vi "ROS_Read_Cam.vi"(8 "error in (no error)":errorcluster, 11 "ROS in":T1) -> (0 "error out":errorcluster, 2 "number":u8[](array[numeric]), 3 "Header":T3)   [LabVIEW 2017]
uses:
  <vilib>/Tufts CEEO ROS for LabVIEW Software/ROS/Code/SubVIs/_ROSControl.ctl
  <vilib>/Tufts CEEO ROS for LabVIEW Software/ROS/Code/SubVIs/_ROSDirection.ctl
  <vilib>/Tufts CEEO ROS for LabVIEW Software/ROS/MessageParsing/std_msgs/subs/parse_string_scalar.vi
  <vilib>/Tufts CEEO ROS for LabVIEW Software/ROS/MessageParsing/std_msgs/subs/parse_u8_array.vi
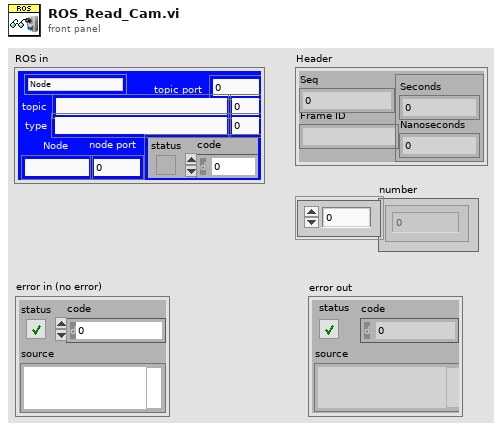
[diagram p1: front panel]
types:
  T1 = typedef "_ROSControl.ctl" = cluster{"topic port":u16, "Node":string, "topic":string, "type":string, "node port":u16, "error ":errorcluster, "Direction":T2, "Update (ms)":u16, "FIFO size":u16}
  T2 = typedef "_ROSDirection.ctl" = enum16{"Node", "Publisher", "Subscriber", "ServiceClient", "ServiceProvider"}
  T3 = cluster{"Seq":u32, "Frame ID":string, "Timestamp":cluster{"Seconds":i32, "Nanoseconds":i32}}
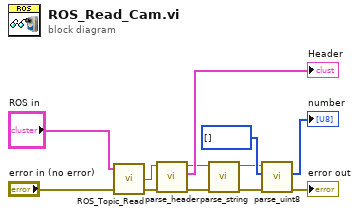
[diagram p0: block diagram]
diagram:
  n1 = call <vilib>:"ROS_Topic_Read.vi"("error in (no error)"="error in (no error)", "ROS in"="ROS in") -> ("error out"=w4:errorcluster, "Reply"=w5:string)  [unwired: 1 in, 1 out]
  n2 = call <vilib>:"parse_header.vi"("error in"=w4, "msg in"=w5) -> ("error out"=w3:errorcluster, "Header"=→"Header":T3, "msg out"=w6:string)  [unwired: 3 in]
  n3 = call-poly <vilib>:"parse_string.vi"("error in"=w3, "msg in"=w6) -> ("error out"=w2:errorcluster, "msg out"=w8:string)  [unwired: 3 in, 1 out]
  n4 = call-poly <vilib>:"parse_uint8.vi"("error in"=w2, "type"=u8[] [], "msg in"=w8) -> ("error out"=→"error out":errorcluster, "number"=→"number":u8[])  [unwired: 2 in, 1 out]
